vi "Auto Comments.vi"() -> (3 "Auto Comment":string)   [LabVIEW 2013]
panel:
  in  "stop":bool
  in  "String":string
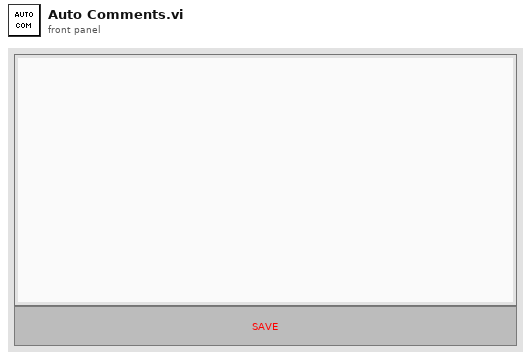
[diagram p1: front panel]
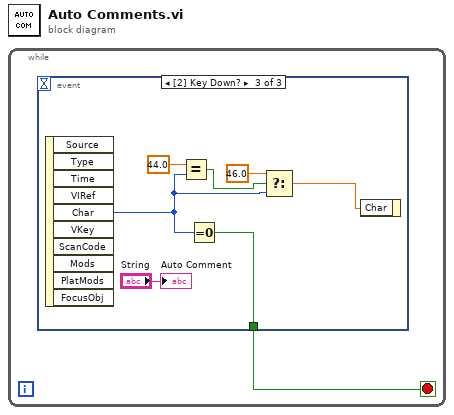
[diagram p0: block diagram]
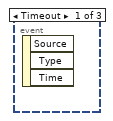
[diagram p2: hidden frame]
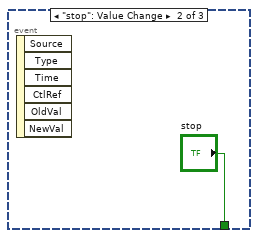
[diagram p3: hidden frame]
diagram:
  n1 = while {
    stop <- w1 stop-if-true
    n2 = event shown="[2] Key Down?" {
      selector: _ -> [_ _ _]
      dyn-events: _ -> [_ _ _]
      timeout: _ -> [_ _ _]
      tunnel: [_ "stop" w3] -> w1
      event Timeout {
        n3 = event-data() -> ()  [unwired: 1 in, 3 out]
      }
      event "stop": Value Change {
        n4 = event-data() -> ()  [unwired: 1 in, 6 out]
      }
      event Key Down? {
        n5 = event-data() -> ("Char"=w4:i16)  [unwired: 1 in, 9 out]
        n6 = Equal?(x=44.0, y=w4) -> (x = y?=w7:bool)
        n7 = Equal To 0?(x=w4) -> (x = 0?=w3:bool)
        n8 = Select(t=46.0, s=w7, f=w4) -> (s? t:f=w6:dbl)
        n9 = event-data("Char"=w6) -> ()  [unwired: 1 in, 1 out]
        "Auto Comment" <- "String"
      }
    }
  }
